vi "Read PIDs.vi"(8 "error in (no error)":errorcluster, 10 "PID Sections to read":string[](array[string]), 11 "FileConfig in":refnum<class "FileConfig.lvclass">) -> (0 "error out":errorcluster, 1 "Found?":bool, 2 "PIDF Array":T1[](array[typedef]), 3 "FileConfig out":refnum<class "FileConfig.lvclass">)   [LabVIEW 2018, in "Config.lvlib" / "FileConfig.lvclass"]
uses:
  FileConfig.lvclass
  <vilib>/Rock Robotics/WPI/ThirdParty/Phoenix-LabVIEW/Motor Controller/Controls/CTRE_Phoenix_MotorControl_SlotStructure.ctl
  Config/Controls/KeyType.ctl
  Config.lvclass
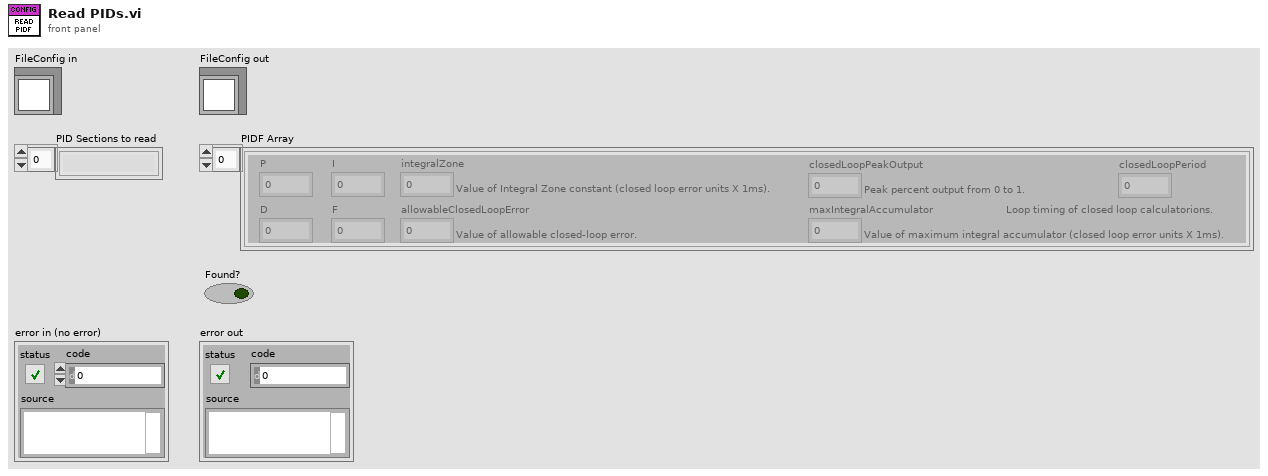
[diagram p1: front panel]
types:
  T1 = typedef "CTRE_Phoenix_MotorControl_SlotStructure.ctl" = cluster{"P":dbl, "I":dbl, "D":dbl, "F":dbl, "integralZone":dbl, "allowableClosedLoopError":i32, "maxIntegralAccumulator":dbl, "closedLoopPeakOutput":dbl, "closedLoopPeriod":i32}
  T2 = typedef "Config.lvlib/Config.lvclass/KeyType.ctl" = enum16{"dbl", "path", "string ", "u32", "i32", "boolean"}
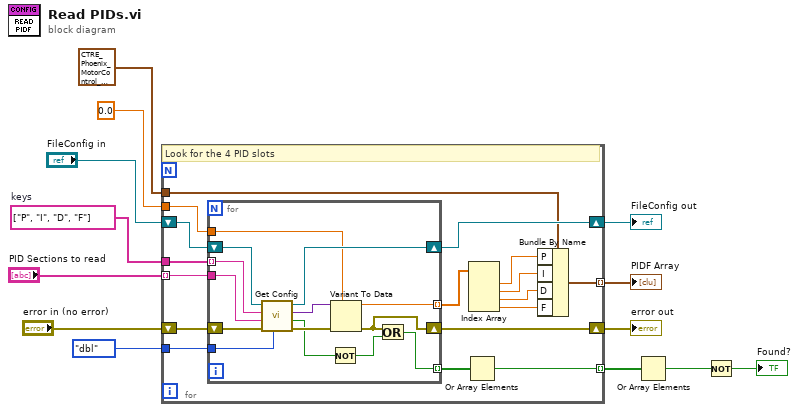
[diagram p0: block diagram]
diagram:
  w6 = string[] ["P", "I", "D", "F"]  # keys
  n1 = for {
    tunnel: 0.0 -> [w26]
    tunnel: KeyType."dbl" -> [w25]
    tunnel: w6 -> [w24]
    shift-right: [w29] -> w11
    shift-left: "FileConfig in" -> [w30]
    shift-right: [w27] -> w3
    shift-left: "error in (no error)" -> [w28]
    tunnel: "PID Sections to read" -> [w23] mode=indexing
    tunnel: [w21] -> w9 mode=indexing
    tunnel: T1 {"P"=0.0, "I"=0.0, "D"=0.0, "F"=0.0, "integralZone"=0.0, "allowableClosedLoopError"=0, "maxIntegralAccumulator"=0.0, "closedLoopPeakOutput"=1.0, "closedLoopPeriod"=1} ("PID Slot 0") -> [w19]
    tunnel: [w18] -> w12 mode=indexing
    # "Look for the 4 PID slots"
    n2 = for {
      shift-right: [w43] -> w29
      shift-left: w30 -> [w44]
      shift-right: [w35] -> w27
      shift-left: w28 -> [w42]
      tunnel: w24 -> [w40] mode=indexing
      tunnel: w25 -> [w39]
      tunnel: w26 -> [w37]
      tunnel: [w36] -> w20 mode=indexing
      tunnel: [w32] -> w22 mode=indexing
      tunnel: w23 -> [w31]
      n3 = call-dynamic "Get Config.vi"(6:w39, "error in (no error)"=w42, "section"=w31, "key"=w40, "FileConfig in"=w44) -> ("error out"=w41:errorcluster, "found?"=w34:bool, "Data"=w38:variant, "FileConfig out"=w43:refnum<class "FileConfig.lvclass">)  [unwired: 3 in]
      n4 = Not(x=w34) -> (.not. x?=w33:bool)
      n5 = Variant To Data(error in=w41, type=w37, Variant=w38) -> (data=w36:dbl, error out=w35:errorcluster)
      n6 = Or(x=w35, y=w33) -> (x .or. y?=w32:bool)
    }
    n7 = Or Array Elements(Boolean array=w22) -> (logical OR=w21:bool)
    n8 = Index Array(array=w20) -> (element #1=w17:dbl, element #2=w16:dbl, element #3=w15:dbl, element #4=w14:dbl)  [unwired: 4 in]
    n9 = Bundle By Name(cluster=w19, "P"=w17, "I"=w16, "D"=w15, "F"=w14) -> (w18:T1)
  }
  "PIDF Array" <- w12
  "FileConfig out" <- w11
  "error out" <- w3
  n10 = Or Array Elements(Boolean array=w9) -> (logical OR=w10:bool)
  n11 = Not(x=w10) -> (.not. x?=→"Found?":bool)
